vi "About.A_Propos_d'elc.vi"   [LabVIEW 2020]
doc: "Fenêtre de présentation du logiciel\nIHM&GTBF32xx\npar Paul GABION"
uses:
  <vilib>/Utility/miscctls.llb/LVPointTypeDef.ctl
panel:
  # "This product uses the following technologies licensed under the corresponding licenses."
  # "(c) 2005-2018 National Instruments.  ALL RIGHTS RESERVED."
  # "ALR32xx Programme élémentaire"
  # "VERSION 1.6.0"
  # "Développé sous LabView 2020\npar Paul GABION"
  # "© 2008-2020 elc  ALL RIGHTS RESERVED."
  # "This product is licensed to you by National Instruments pursuant \nto the applicable National Instruments software license agreement."
types:
  T1 = typedef "LVPointTypeDef.ctl" = cluster{"Horizontal":i16, "Vertical":i16}
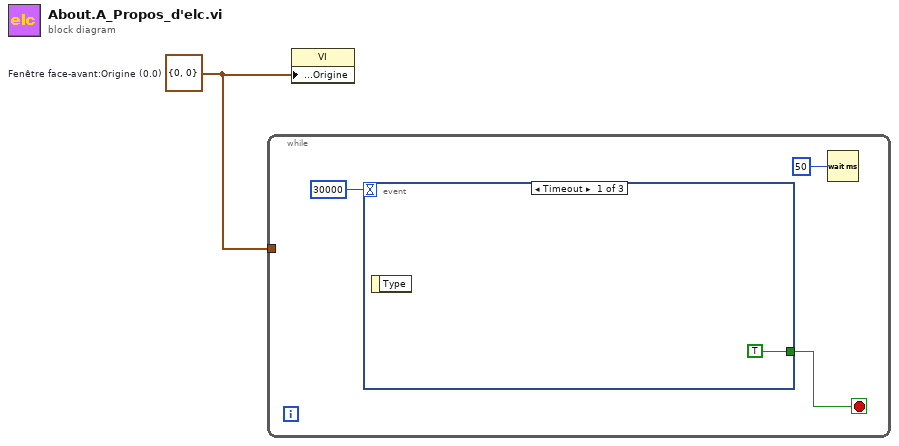
[diagram p0: block diagram]
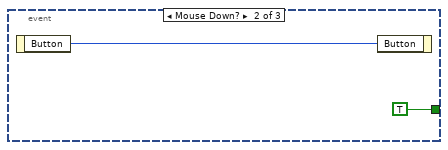
[diagram p2: hidden frame]
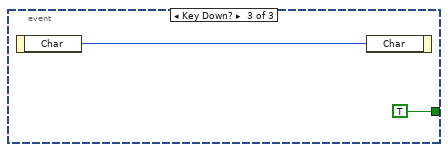
[diagram p3: hidden frame]
diagram:
  w1 = T1 {"Horizontal"=0, "Vertical"=0}  # Fenêtre face-avant:Origine (0.0)
  n1 = while {
    tunnel: w1 -> [_]
    stop <- w3 stop-if-true
    n2 = event shown="[0] Timeout" {
      selector: _ -> [_ _ _]
      dyn-events: _ -> [_ _ _]
      timeout: 30000 -> [_ _ _]
      tunnel: [TRUE TRUE TRUE] -> w3
      event Timeout {
        n3 = event-data() -> ()  [unwired: 1 in, 1 out]
      }
      event Mouse Down? {
        n4 = event-data() -> ("Button"=w6:u16)  [unwired: 1 in]
        n5 = event-data("Button"=w6) -> ()  [unwired: 1 in, 1 out]
      }
      event Key Down? {
        n6 = event-data() -> ("Char"=w8:i16)  [unwired: 1 in]
        n7 = event-data("Char"=w8) -> ()  [unwired: 1 in, 1 out]
      }
    }
    n8 = Wait (ms)(milliseconds to wait=u32 50 ("attente (ms)")) -> ()  [unwired: 1 out]
  }
  n9 = property class="VI"("Fenêtre face-avant:Origine"=w1) -> ()  [unwired: 2 in, 2 out]
